vi "sub_est_noise_power - G1.vi"(8 "Bin Size":i32=100, 10 "Input Complex Samples":cdb[](array[numeric])) -> (0 "Energy Threshold":dbl, 2 "noise_power":dbl, 4 "signal_power":dbl, 5 "noise_estimation_error ?":bool)   [LabVIEW 2013]
panel:
  out "power":dbl[](array[numeric])
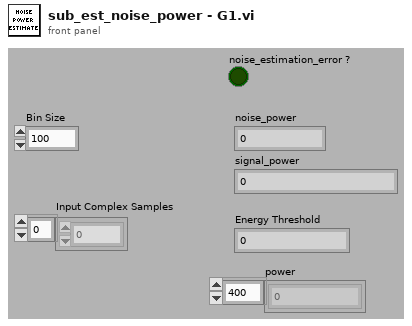
[diagram p1: front panel]
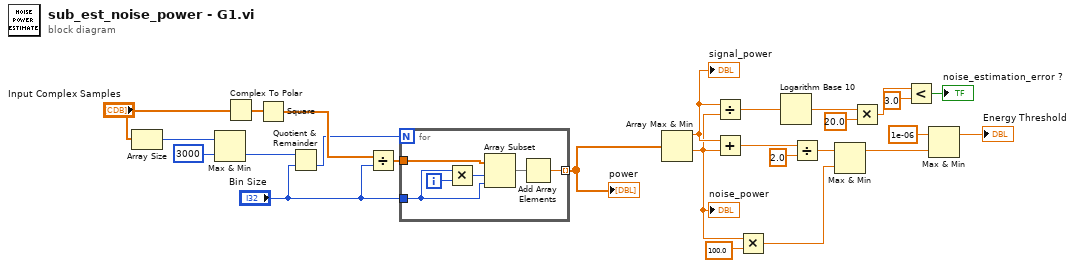
[diagram p0: block diagram]
diagram:
  n1 = Array Size(array="Input Complex Samples") -> (size(s)=w25:i32)
  n2 = Max & Min(x=w25, y=3000) -> (min(x,y)=w24:i32)  [unwired: 1 out]
  n3 = Complex To Polar(r * e^(i*theta)="Input Complex Samples") -> (r=w5:dbl[])  [unwired: 1 out]
  n4 = Square(x=w5) -> (x^2=w4:dbl[])
  n5 = Quotient & Remainder(x=w24, y="Bin Size") -> (floor(x/y)=w2:i32)  [unwired: 1 out]
  n6 = Divide(x=w4, y="Bin Size") -> (x/y=w3:dbl[])
  n7 = for {
    N: w2 -> [_]
    tunnel: w3 -> [w32]
    tunnel: "Bin Size" -> [w28]
    tunnel: [w31] -> w22 mode=indexing
    i -> [w30]
    n8 = Multiply(x=w28, y=w30) -> (x*y=w29:i32)
    n9 = Array Subset(array=w32, index=w29, length=w28) -> (w27:dbl[])
    n10 = Add Array Elements(numeric array=w27) -> (sum=w31:dbl)
  }
  "power" <- w22
  n11 = Array Max & Min(array=w22) -> (max value=w15:dbl, min value=w11:dbl)  [unwired: 2 out]
  "noise_power" <- w11
  "signal_power" <- w15
  n12 = Divide(x=w15, y=w11) -> (x/y=w21:dbl)
  n13 = Add(x=w15, y=w11) -> (x+y=w14:dbl)
  n14 = Multiply(x=w11, y=100.0) -> (x*y=w9:dbl)
  n15 = Logarithm Base 10(1:w21) -> (0:w20:dbl)
  n16 = Divide(x=w14, y=2.0) -> (x/y=w12:dbl)
  n17 = Max & Min(x=w12, y=w9) -> (max(x,y)=w8:dbl)  [unwired: 1 out]
  n18 = Multiply(x=w20, y=20.0) -> (x*y=w18:dbl)
  n19 = Less?(x=w18, y=3.0) -> (x < y?=→"noise_estimation_error ?":bool)
  n20 = Max & Min(x=1e-06 ("y"), y=w8) -> (max(x,y)=→"Energy Threshold":dbl)  [unwired: 1 out]
